vi "Add DataTable To DataSet.vi"(8 "错误输入（无错误）":errorcluster, 10 "DataTable":refnum<k24>, 11 "DataSet In":refnum<k24>) -> (0 "错误输出":errorcluster, 3 "DataSet Out":refnum<k24>)   [LabVIEW 2012, in "DataGridView.lvlib"]
uses:
  DataGridView.lvlib
  System.Data
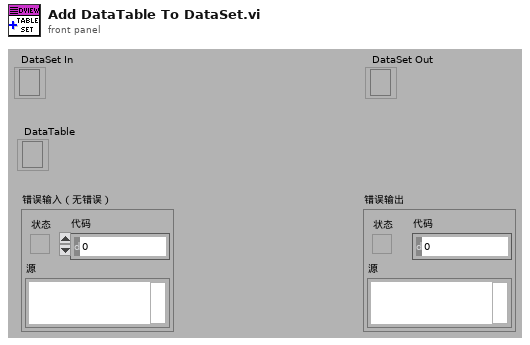
[diagram p1: front panel]
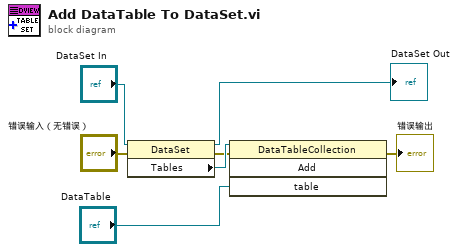
[diagram p0: block diagram]
diagram:
  n1 = property class="DataSet"(reference="DataSet In", error in="错误输入（无错误）") -> (reference out=→"DataSet Out":refnum<k24>, error out=w5:errorcluster, "Tables"=w6:refnum<k24>)
  n2 = invoke class="DataTableCollection" method="Add"(reference=w6, error in=w5, "table"="DataTable") -> (error out=→"错误输出":errorcluster)  [unwired: 1 in, 3 out]
